vi "Pass Fail Result Colors.vi"() -> ()   [LabVIEW 2014]
panel:
  in  "NA":u32(colorbox)
  in  "Fail":u32(colorbox)=16719378
  in  "Pass":u32(colorbox)=65379
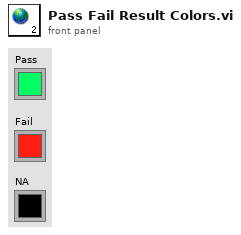
[diagram p1: front panel]
diagram:
